vi "mainstructure.vi"() -> ()   [LabVIEW 2020]
uses:
  <userlib>/Nanonis Prog Interface V5/Nanonis Prog Interface.lvlib
panel:
  in  "Speed (m/s)":sgl=2.066e-07 format="%.2p"
  in  "Bias (V)":sgl=0.5 format="%_5p"
  in  "Z Controller setpoint":sgl=5e-10 format="%#_6p"
  in  "Numeric 2":i32=50
  in  "y":sgl=9.7e-08
  in  "Error in (no error)":errorcluster
  in  "Numeric":i32=50
  out "appended array":sgl[](array[numeric])
  in  "x":sgl=4.45e-07
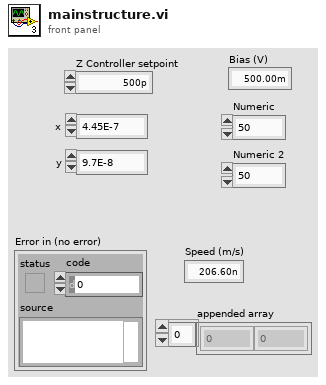
[diagram p1: front panel]
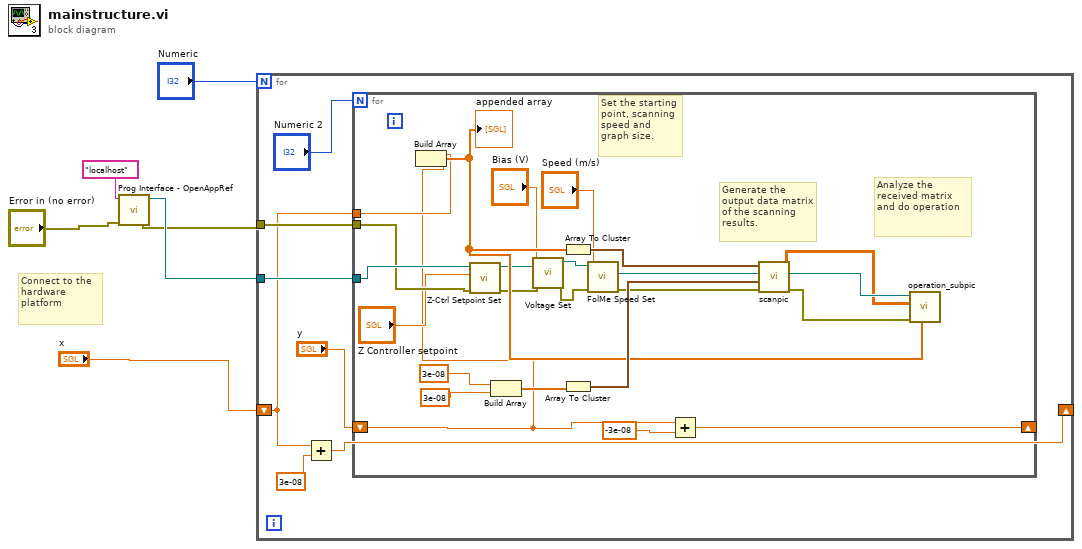
[diagram p0: block diagram]
diagram:
  # "Connect to the hardware platform"
  n1 = call <userlib>:"Prog Interface - OpenAppRef.vi"("Error in (no error)"="Error in (no error)", "Machine name (local machine IP)"="localhost" ("Machine name (localhost)")) -> ("Error out"=w2:errorcluster, "Application reference"=w3:refnum<vi>)  [unwired: 4 in]
  n2 = for {
    N: "Numeric" -> [_]
    shift-right: [w10] -> _
    shift-left: "x" -> [w9]
    tunnel: w3 -> [w13]
    tunnel: w2 -> [w12]
    n3 = Add(x=w9, y=3e-08) -> (x+y=w10:dbl)
    n4 = for {
      N: "Numeric 2" -> [_]
      shift-right: [w27] -> _
      shift-left: "y" -> [w14]
      tunnel: w13 -> [w25]
      tunnel: w12 -> [w24]
      tunnel: w9 -> [w26]
      # "Analyze the received matrix and do operation"
      # "Generate the output data matrix of the scanning results."
      # "Set the starting point, scanning speed and graph size."
      n5 = Build Array(w26, w14) -> (w29:dbl[])
      "appended array" <- w29
      n6 = call <userlib>:"Z-Ctrl Setpoint Set.vi"("error in (no error)"=w24, "Z Controller setpoint"="Z Controller setpoint", "Application ref in"=w25) -> ("error out"=w22:errorcluster, "Application ref out"=w21:refnum<vi>)  [unwired: 7 in]
      n7 = Build Array(3e-08 ("element"), 3e-08 ("element")) -> (w32:dbl[])
      n8 = call <userlib>:"Voltage Set.vi"("Error in (no error)"=w22, "Bias (V)"="Bias (V)", "Application ref in"=w21) -> ("Error out"=w18:errorcluster, "Application ref out"=w19:refnum<vi>)  [unwired: 7 in]
      n9 = Array To Cluster(array=w29) -> (cluster=w37:cluster{"[0]":dbl, "[1]":dbl})
      n10 = Array To Cluster(array=w32) -> (cluster=w33:cluster{"[0]":dbl, "[1]":dbl})
      n11 = call <userlib>:"FolMe Speed Set.vi"("error in (no error)"=w18, "Speed (m/s)"="Speed (m/s)", "Application ref in"=w19) -> ("error out"=w17:errorcluster, "Application ref out"=w16:refnum<vi>)  [unwired: 5 in]
      n12 = Add(x=w14, y=-3e-08) -> (x+y=w27:dbl)
      n13 = call "scanpic.vi"("error in (no error)"=w17, "Size (m)"=w33, "Application ref in"=w16, "Center coordinates (m)"=w37) -> ("Error out"=w34:errorcluster, "Application ref out"=w36:refnum<vi>, "Data"=w35:sgl[][])  [unwired: 5 in]
      n14 = call "operation_subpic.vi"("Center Point"=w29, "error in (no error)"=w34, "XYData"=w35, "Application ref in"=w36) -> ()  [unwired: 8 in]
    }
  }
